vi "Errors.vi"   [LabVIEW 2017, in "DSF Core.lvlib" / "Transfer Group.lvclass"]
uses:
  Transfer Group/Transfer Group.lvclass
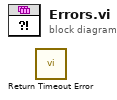
[diagram p0: block diagram]
diagram:
  n1 = call "Return Timeout Error.vi"() -> ()  [unwired: 10 in, 2 out]
